vi "ATE_Test_Pulse.vi"() -> ()   [LabVIEW 2009]
doc: "Use this template to build a producer/consumer design pattern with events to produce queue items. Use this design pattern instead of the User Interface Event Handler pattern for user interfaces when you want to execute code asynchronously in response to an event without slowing the user interface responsiveness."
panel:
  in  "exit":bool
  in  "ATE TP TABS":enum32{"SPOL Test Pulse Control and Status"}(tab)
  in  "Signal Generator Control":T1={"Frequency (GHz)"=2.809, "RF Power (dBm)"=-120.0, "RF ON/OFF"=FALSE} {"RF Power (dBm)" min=-120.0 max=20.0 step=5.0 format="%.2g"; "Frequency (GHz)" min=0.6 max=3.0 step=0.001 format="%#_9g"}
  out "Signal Generator Status":T2={"Frequency (GHz)"=2.809, "RF Power (dBm)"=-120.0, "RF Power"=FALSE} {"RF Power (dBm)" format="%.2g"}
  out "Switch Position\nVerfied":bool
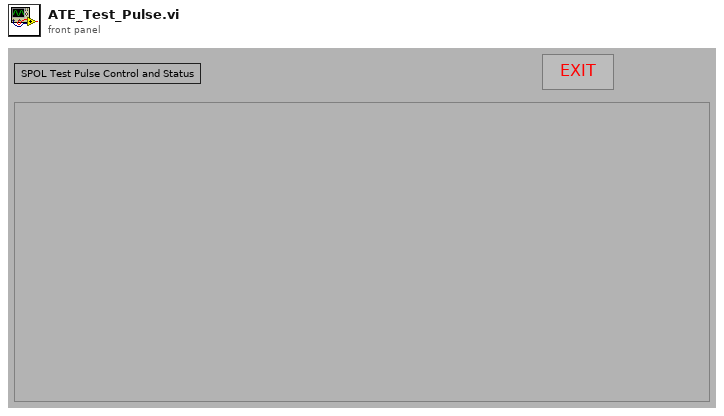
[diagram p1: front panel]
types:
  T1 = cluster{"Frequency (GHz)":dbl, "RF Power (dBm)":dbl, "RF ON/OFF":bool}
  T2 = cluster{"Frequency (GHz)":dbl, "RF Power (dBm)":dbl, "RF Power":bool}
  T3 = enum16{"NONE", "Amp Bypass Switch", "Test Pulse Generator", "Power Meter Switch (S5)"}
  T4 = enum16{"NONE", "Delay Device", "Signal Generator (J7)", "Inside Noise Box NF (J5)", "2W Term (TM3)"}
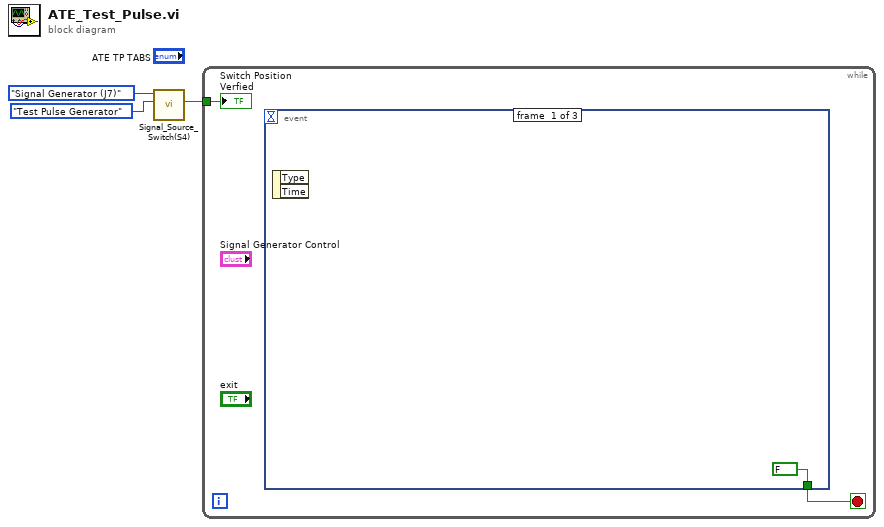
[diagram p0: block diagram]
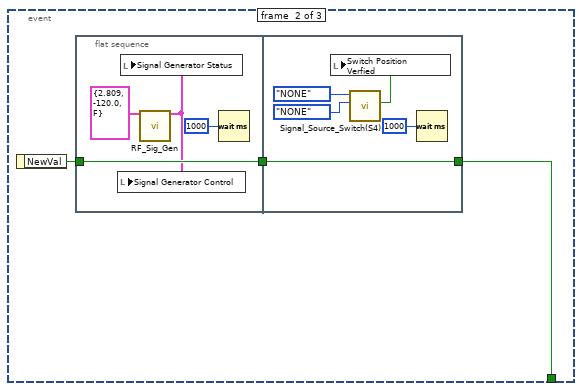
[diagram p2: hidden frame]
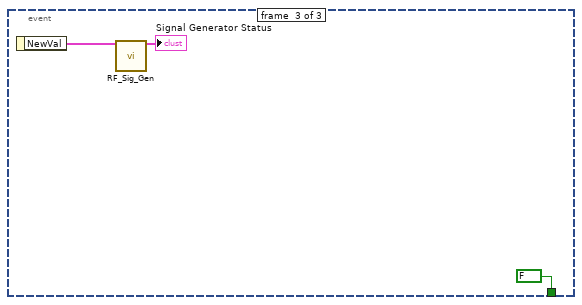
[diagram p3: hidden frame]
diagram:
  n1 = call "Signal_Source_Switch(S4).vi"("Output"=T3."Test Pulse Generator" ("ATE Switch (S4) Output"), "Input"=T4."Signal Generator (J7)" ("ATE Switch (S4) Input")) -> ("Verfied"=w1:bool)  [unwired: 7 in, 2 out]
  n2 = while {
    tunnel: w1 -> [w4]
    stop <- w5 stop-if-true
    n3 = event shown="[1] \"exit\": Value Change" {
      selector: _ -> [_ _ _]
      dyn-events: _ -> [_ _ _]
      timeout: _ -> [_ _ _]
      tunnel: [FALSE w9 FALSE] -> w5
      event #0 {
        n4 = event-data() -> ()  [unwired: 1 in, 2 out]
      }
      event #1 {
        n5 = event-data() -> ("NewVal"=w8:bool)  [unwired: 1 in]
        n6 = flat-sequence {
          tunnel: w8 -> [w11]
          tunnel: [w11] -> w7
          tunnel: [w14] -> w9
          tunnel: w7 -> [w14]
          frame #0 {
            n7 = call "RF_Sig_Gen.vi"("Signal Generator Control"=T1 {"Frequency (GHz)"=2.809, "RF Power (dBm)"=-120.0, "RF ON/OFF"=FALSE}) -> ("Signal Generator Status"=w10:T2)  [unwired: 13 in, 1 out]
            n8 = local write "Signal Generator Control"(w10) -> ()
            n9 = local write "Signal Generator Status"(w10) -> ()
            n10 = Wait (ms)(milliseconds to wait=u32 1000) -> ()  [unwired: 1 out]
          }
          frame #1 {
            n11 = call "Signal_Source_Switch(S4).vi"("Output"=T3."NONE" ("ATE Switch (S4) Output"), "Input"=T4."NONE" ("ATE Switch (S4) Input")) -> ("Verfied"=w18:bool)  [unwired: 7 in, 2 out]
            n12 = local write "Switch Position\nVerfied"(w18) -> ()
            n13 = Wait (ms)(milliseconds to wait=u32 1000) -> ()  [unwired: 1 out]
          }
        }
      }
      event #2 {
        n14 = event-data() -> ("NewVal"=w20:T1)  [unwired: 1 in]
        n15 = call "RF_Sig_Gen.vi"("Signal Generator Control"=w20) -> ("Signal Generator Status"=→"Signal Generator Status":T2)  [unwired: 13 in, 1 out]
      }
    }
    "Switch Position\nVerfied" <- w4
  }
